vi "Teleop.vi"(10 "Match Info":T1={"Autonomous Elapsed Seconds"=0.0, "TeleOp Elapsed Seconds"=0.0, "Disabled Elapsed Seconds"=0.0, "Visited Autonomous"=FALSE, "Visited TeleOp"=FALSE, "Visited Disabled"=FALSE, "Autonomous Settings"={"Autonomous Style"=enum."Independent", "VI Refnum"=refnum}}, 11 "Call Context":T2) -> ()   [LabVIEW 2018]
doc: "This VI is called for each TeleOp packet received from the DS where the robot is not disabled. It is often used to read from the joysticks and update I/O or to update setpoints for timed control loops. It should complete and return within 20 milliseconds or it may miss DS packets."
uses:
  <vilib>/Rock Robotics/WPI/DriverStation/WPI_DriverStationDerivedRobotMode.ctl
  <vilib>/Rock Robotics/WPI/DriverStation/WPI_DriverStationMatch Info.ctl
  <vilib>/Rock Robotics/WPI/Solenoid/WPI_SolenoidValue.ctl
  <vilib>/Rock Robotics/WPI/ThirdParty/Phoenix-LabVIEW/Motor Controller/Controls/CTRE_Phoenix_MotorControl_ControlMode.ctl
  <vilib>/Rock Robotics/WPI/Utilities/WPI_GetSetVariantRefNum.vi
  <vilib>/Rock Robotics/Network Tables/NT Write Boolean Array.vi
  <vilib>/Rock Robotics/Network Tables/NT Write Numeric Array.vi
  <vilib>/Rock Robotics/WPI/Solenoid/WPI_SolenoidSetEnum.vi
  <vilib>/Rock Robotics/Network Tables/NT Read Boolean.vi
  <vilib>/Rock Robotics/Network Tables/NT Read Number.vi
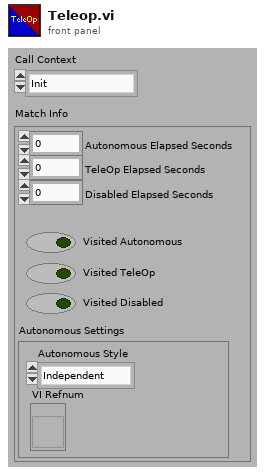
[diagram p1: front panel]
types:
  T1 = typedef "WPI_DriverStationMatch Info.ctl" = cluster{"Autonomous Elapsed Seconds":dbl, "TeleOp Elapsed Seconds":dbl, "Disabled Elapsed Seconds":dbl, "Visited Autonomous":bool, "Visited TeleOp":bool, "Visited Disabled":bool, "Autonomous Settings":cluster{"Autonomous Style":enum16{"Iterative", "Independent"}, "VI Refnum":refnum<vi>}}
  T2 = typedef "WPI_DriverStationDerivedRobotMode.ctl" = enum16{"Init", "Execute", "Stop"}
  T3 = typedef "CTRE_Phoenix_MotorControl_ControlMode.ctl" = u16
  T4 = typedef "WPI_SolenoidValue.ctl" = enum16{"Off", "On", "Forward", "Reverse"}
  T5 = typedef "WPI_JoystickDevRef.ctl" = cluster{"Device":T6}
  T6 = typedef "WPI_JoystickDeviceEnum.ctl" = enum16{"USB 0", "USB 1", "USB 2", "USB 3", "USB 4", "USB 5"}
  T7 = typedef "WPI_MotorControlDeviceRef.ctl" = cluster{"DeviceStatus":errorcluster, "Type":T8, "PWM":cluster{"PWM Channel":T9, "DeadBand":T10}, "CAN":cluster{"Device Number":u8, "SetOutput VI Ref":variant, "GetOutput VI Ref":variant, "Enable VI Ref":variant, "Disable VI Ref":variant, "Data":variant}, "Invert":bool, "DIO PWM":cluster{"PWM \"Enable\" Channel":T9, "DIOChannel":T11, "PWM Rate":dbl}}
  T8 = typedef "WPI_MotorControlType.ctl" = enum16{"PWM", "CAN", "DIO PWM"}
  T9 = typedef "FPGA_DIOPWMChannel.ctl" = enum8{"PWM 0", "PWM 1", "PWM 2", "PWM 3", "PWM 4", "PWM 5", "PWM 6", "PWM 7", "PWM 8", "PWM 9", "PWM MXP 0", "PWM MXP 1", "PWM MXP 2", "PWM MXP 3", "PWM MXP 4", "PWM MXP 5", "PWM MXP 6", "PWM MXP 7", "PWM MXP 8", "PWM MXP 9", "Invalid"}
  T10 = typedef "WPI_PWMDeadband.ctl" = cluster{"Name":string, "maxPositivePwm":i32, "minPositivePwm":i32, "centerPwm":i32, "maxNegativePwm":i32, "minNegativePwm":i32, "angularRange":u16}
  T11 = typedef "FPGA_DIOChannel.ctl" = enum8{"DIO 0", "DIO 1", "DIO 2", "DIO 3", "DIO 4", "DIO 5", "DIO 6", "DIO 7", "DIO 8", "DIO 9", "DIO MXP 0", "DIO MXP 1", "DIO MXP 2", "DIO MXP 3", "DIO MXP 4", "DIO MXP 5", "DIO MXP 6", "DIO MXP 7", "DIO MXP 8", "DIO MXP 9", "DIO MXP 10", "DIO MXP 11", "DIO MXP 12", "DIO MXP 13", "DIO MXP 14", "DIO MXP 15", "SPI Port CS1", "SPI Port CS2", "SPI Port CS3", "SPI Port MISO", "SPI Port MOSI", "Invalid"}
  T12 = typedef "WPI_SolenoidDevRef.ctl" = cluster{"DevStatus":errorcluster, "Pneumatics Control Module":u8, "Forward Solenoid Channel":T13, "Reverse Solenoid Channel":T13}
  T13 = typedef "WPI_SolenoidChannel.ctl" = enum8{"Solenoid 0", "Solenoid 1", "Solenoid 2", "Solenoid 3", "Solenoid 4", "Solenoid 5", "Solenoid 6", "Solenoid 7", "Invalid"}
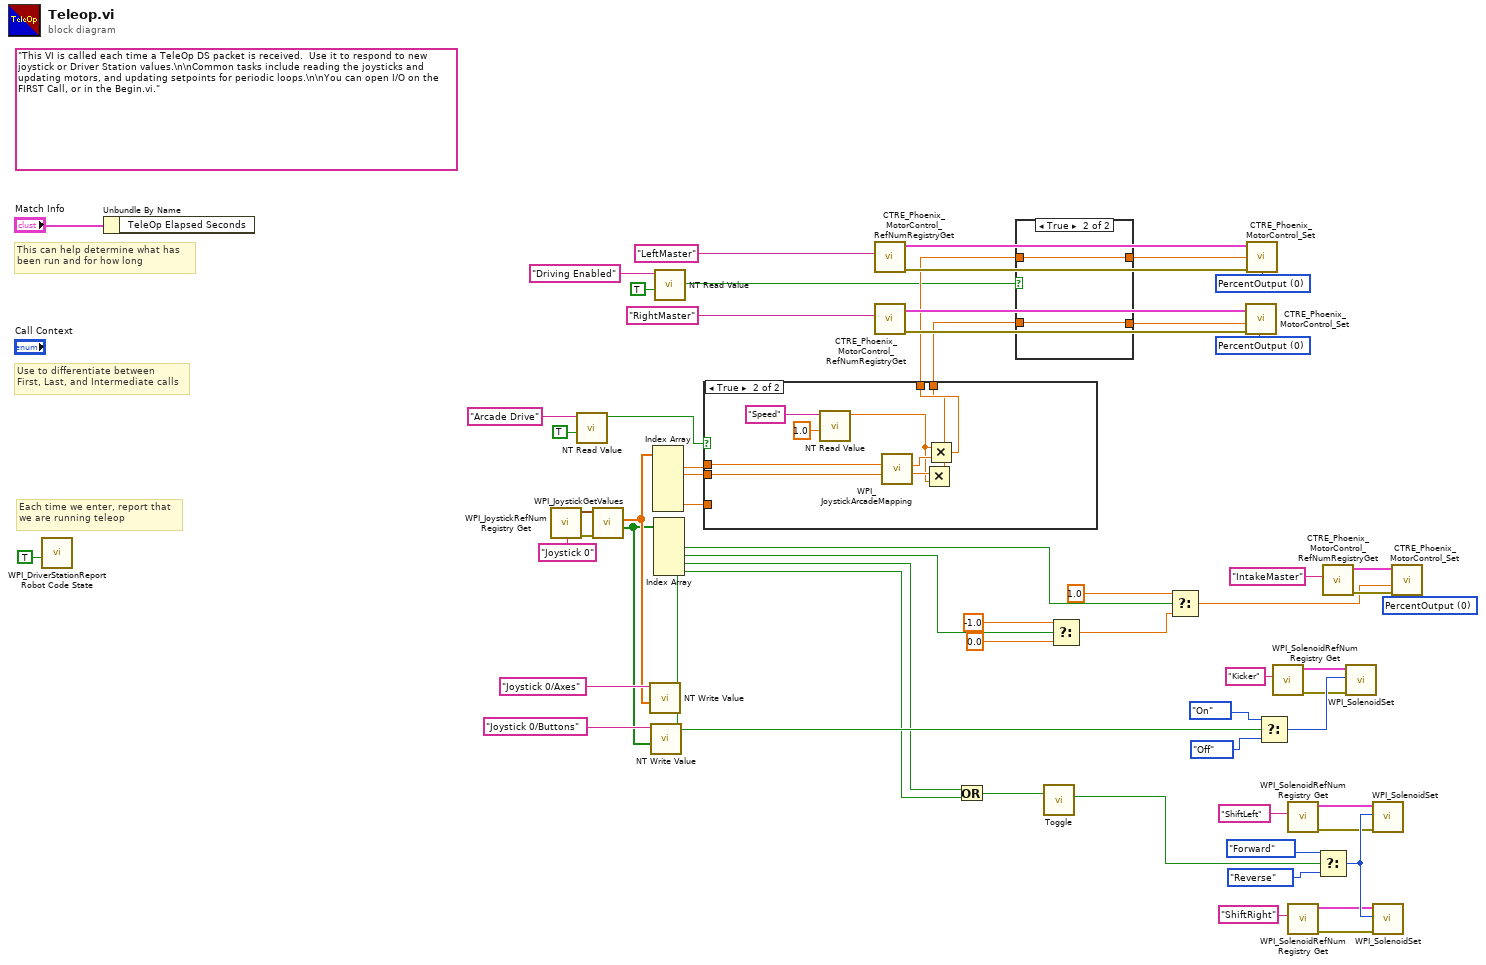
[diagram p0: block diagram]
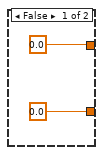
[diagram p3: hidden frame]
diagram:
  w21 = T3 0 items=["PercentOutput"=0, "Position"=1, "Velocity"=2, "Current"=3, "Follower"=5, "MotionProfile"=6, "MotionMagic"=7, "MotionProfileArc"=10, "Disabled"=15] ("Control Mode")
  w36 = T3 0 items=["PercentOutput"=0, "Position"=1, "Velocity"=2, "Current"=3, "Follower"=5, "MotionProfile"=6, "MotionMagic"=7, "MotionProfileArc"=10, "Disabled"=15] ("Control Mode")
  w37 = T3 0 items=["PercentOutput"=0, "Position"=1, "Velocity"=2, "Current"=3, "Follower"=5, "MotionProfile"=6, "MotionMagic"=7, "MotionProfileArc"=10, "Disabled"=15] ("Control Mode")
  (unwired) "This VI is called each time a TeleOp DS packet is received.  Use it to respond to new joystick or Driver Station values.\n\nCommon tasks include reading the joysticks and updating motors, and updating setpoints for periodic loops.\n\nYou can open I/O on the FIRST Call, or in the Begin.vi."
  # "Each time we enter, report that\nwe are running teleop"
  # "Use to differentiate between\nFirst, Last, and Intermediate calls"
  # "This can help determine what has\nbeen run and for how long"
  n1 = call <vilib>:"WPI_DriverStationReport Robot Code State.vi"("TeleOp"=TRUE ("Autonomous")) -> ()  [unwired: 10 in, 1 out]
  n2 = Unbundle By Name("Match Info") -> ()  [unwired: 1 out]
  n3 = call <vilib>:"WPI_JoystickRefNum Registry Get.vi"("refnum name"="Joystick 0") -> ("error out"=w27:errorcluster, "JoystickDevRef"=w59:T5)  [unwired: 1 in, 8 out]
  n4 = call-poly <vilib>:"NT Read Value.vi"("Default Value"=TRUE, "Name"="Arcade Drive") -> ("Boolean"=w5:bool)  [unwired: 8 in, 1 out]
  n5 = call <vilib>:"WPI_JoystickGetValues.vi"("error in (no error)"=w27, "JoystickDevRef"=w59) -> ("Buttons"=w50:bool[], "Axes"=w55:dbl[])  [unwired: 5 in, 3 out]
  n6 = call-poly <vilib>:"NT Write Value.vi"("Numeric Array"=w55, "Name"="Joystick 0/Axes") -> ()  [unwired: 9 in, 1 out]
  n7 = call-poly <vilib>:"NT Write Value.vi"("Boolean Array"=w50, "Name"="Joystick 0/Buttons") -> ()  [unwired: 9 in, 1 out]
  n8 = Index Array(array=w55) -> (element #1=w10:dbl, element #2=w9:dbl, element #6=w8:dbl)  [unwired: 6 in, 3 out]
  n9 = Index Array(array=w50) -> (element #1=w49:bool, element #2=w18:bool, element #3=w16:bool, element #4=w22:bool, element #5=w23:bool)  [unwired: 5 in]
  n10 = call-poly <vilib>:"NT Read Value.vi"("Default Value"=TRUE, "Name"="Driving Enabled") -> ("Boolean"=w11:bool)  [unwired: 8 in, 1 out]
  n11 = case shown="True" w5 {
    tunnel: w10 -> [_ w72]
    tunnel: w9 -> [w63 w71]
    tunnel: [w63 w68] -> w32
    tunnel: [w62 w67] -> w30
    tunnel: w8 -> [w62 _]
    frame False {
    }
    frame True {
      n12 = call-poly <vilib>:"NT Read Value.vi"("Default Value"=1.0, "Name"="Speed") -> ("Numeric"=w64:dbl)  [unwired: 8 in, 1 out]
      n13 = call <vilib>:"WPI_JoystickArcadeMapping.vi"("Y axis value"=w71, "X axis value"=w72) -> ("Right Motor Value"=w69:dbl, "Left Motor Value"=w70:dbl)  [unwired: 8 in]
      n14 = Multiply(x=w69, y=w64) -> (x*y=w67:dbl)
      n15 = Multiply(x=w64, y=w70) -> (x*y=w68:dbl)
    }
  }
  n16 = call <vilib>:"CTRE_Phoenix_MotorControl_RefNumRegistryGet.vi"("refnum name"="LeftMaster") -> ("error out"=w35:errorcluster, "PhoenixMotorControlDevRef"=w52:T7)  [unwired: 9 in]
  n17 = call <vilib>:"CTRE_Phoenix_MotorControl_RefNumRegistryGet.vi"("refnum name"="RightMaster") -> ("error out"=w34:errorcluster, "PhoenixMotorControlDevRef"=w51:T7)  [unwired: 9 in]
  n18 = Or(x=w22, y=w23) -> (x .or. y?=w40:bool)
  n19 = case shown="True" w11 {
    tunnel: [0.0 w76] -> w33
    tunnel: w32 -> [_ w76]
    tunnel: [0.0 w75] -> w31
    tunnel: w30 -> [_ w75]
    frame False {
    }
    frame True {
    }
  }
  n20 = call "Toggle.vi"("Input"=w40) -> ("Output"=w39:bool)  [unwired: 10 in]
  n21 = Select(t=-1.0, s=w16, f=0.0) -> (s? t:f=w17:dbl)
  n22 = Select(t=1.0, s=w18, f=w17) -> (s? t:f=w12:dbl)
  n23 = call <vilib>:"CTRE_Phoenix_MotorControl_Set.vi"("error in (no error)"=w34, "Output"=w31, "Control Mode"=w36, "PhoenixMotorControlDevRef"=w51) -> ()  [unwired: 6 in, 2 out]
  n24 = call <vilib>:"CTRE_Phoenix_MotorControl_Set.vi"("error in (no error)"=w35, "Output"=w33, "Control Mode"=w37, "PhoenixMotorControlDevRef"=w52) -> ()  [unwired: 6 in, 2 out]
  n25 = Select(t=WPI_SolenoidValue."On" ("Value"), s=w49, f=WPI_SolenoidValue."Off") -> (s? t:f=w45:T4)
  n26 = call <vilib>:"WPI_SolenoidRefNum Registry Get.vi"("refnum name"="Kicker") -> ("error out"=w25:errorcluster, "SolenoidDevRef"=w44:T12)  [unwired: 9 in]
  n27 = call <vilib>:"WPI_SolenoidRefNum Registry Get.vi"("refnum name"="ShiftLeft") -> ("error out"=w26:errorcluster, "SolenoidDevRef"=w43:T12)  [unwired: 9 in]
  n28 = call <vilib>:"WPI_SolenoidRefNum Registry Get.vi"("refnum name"="ShiftRight") -> ("error out"=w1:errorcluster, "SolenoidDevRef"=w2:T12)  [unwired: 9 in]
  n29 = Select(t=WPI_SolenoidValue."Forward" ("Value"), s=w39, f=WPI_SolenoidValue."Reverse") -> (s? t:f=w38:T4)
  n30 = call <vilib>:"CTRE_Phoenix_MotorControl_RefNumRegistryGet.vi"("refnum name"="IntakeMaster") -> ("error out"=w19:errorcluster, "PhoenixMotorControlDevRef"=w20:T7)  [unwired: 9 in]
  n31 = call-poly <vilib>:"WPI_SolenoidSet.vi"("error in (no error)"=w25, "Value"=w45, "SolenoidDevRef"=w44) -> ()  [unwired: 7 in, 2 out]
  n32 = call-poly <vilib>:"WPI_SolenoidSet.vi"("error in (no error)"=w26, "Value"=w38, "SolenoidDevRef"=w43) -> ()  [unwired: 7 in, 2 out]
  n33 = call-poly <vilib>:"WPI_SolenoidSet.vi"("error in (no error)"=w1, "Value"=w38, "SolenoidDevRef"=w2) -> ()  [unwired: 7 in, 2 out]
  n34 = call <vilib>:"CTRE_Phoenix_MotorControl_Set.vi"("error in (no error)"=w19, "Output"=w12, "Control Mode"=w21, "PhoenixMotorControlDevRef"=w20) -> ()  [unwired: 6 in, 2 out]
